vi "使用子VI.vi"() -> ()   [LabVIEW 2021]
doc: "本VI是为《我和LabVIEW》一书编写的示例。\n关于本书的介绍请参考网页：\nhttp://ruanqizhen.spaces.live.com/blog/cns!5852D4F797C53FB6!4310.entry"
panel:
  out "波形图":dbl[](graph)
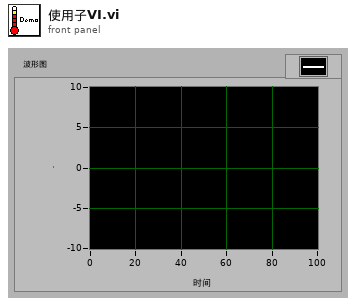
[diagram p1: front panel]
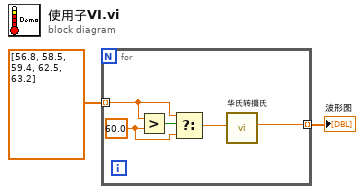
[diagram p0: block diagram]
diagram:
  n1 = for {
    tunnel: dbl[] [56.8, 58.5, 59.4, 62.5, 63.2] -> [w5] mode=indexing
    tunnel: [w7] -> w1 mode=indexing
    w4 = 60.0 ("y")
    n2 = Greater?(x=w5, y=w4) -> (0:w6:bool)
    n3 = Select(t=w5, s=w6, f=w4) -> (s? t:f=w3:dbl)
    n4 = call "华氏转摄氏.vi"("华氏温度"=w3) -> ("摄氏温度"=w7:dbl)  [unwired: 10 in]
  }
  "波形图" <- w1
